vi "Configure Channel Trigger.vi"(6 "Trigger Level (0 V)":dbl, 7 "Units (0: Volt)":i32(ring) items=["Volt", "Ampere"], 8 "error in (no error)":errorcluster, 9 "Vertical Range (8.0 V)":dbl=8.0, 10 "Probe Attenuation Factor (1.0 X)":dbl=1.0, 11 "VISA resource name":refnum<visa-resource-name>) -> (0 "error out":errorcluster, 3 "VISA resource name out":refnum<visa-resource-name>)   [LabVIEW 2023, in "Keysight-DSQx3014T.lvlib"]
doc: "Configures the channel setting for External Trigger."
uses:
  Keysight-DSQx3014T.lvlib
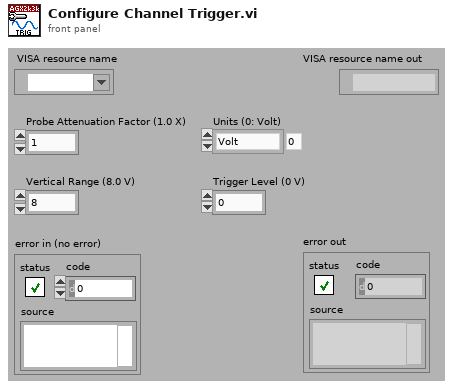
[diagram p1: front panel]
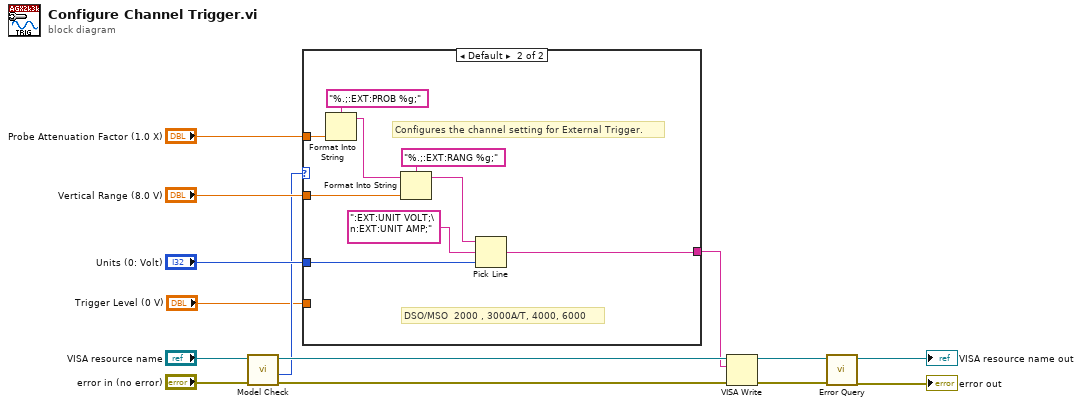
[diagram p0: block diagram]
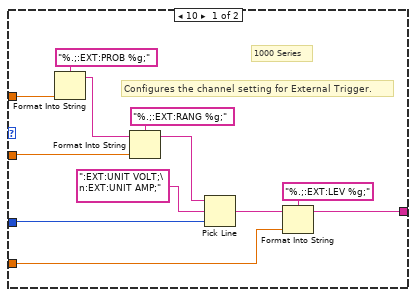
[diagram p2: hidden frame]
diagram:
  n1 = call "Model Check.vi"("error in (no error)"="error in (no error)", "VISA resource name"="VISA resource name") -> ("error out"=w4:errorcluster, "Model"=w2:i32, "VISA resource name out"=w5:refnum<visa-resource-name>)  [unwired: 6 in, 1 out]
  n2 = case shown="Default" w2 {
    tunnel: "Probe Attenuation Factor (1.0 X)" -> [w21 w34]
    tunnel: "Vertical Range (8.0 V)" -> [w20 w31]
    tunnel: "Units (0: Volt)" -> [w19 w29]
    tunnel: [w16 w27] -> w3
    tunnel: "Trigger Level (0 V)" -> [w18 _]
    frame 10 {
      # "1000 Series"
      # "Configures the channel setting for External Trigger."
      n3 = Format Into String(format string="%.;:EXT:PROB %g;", w21) -> (resulting string=w25:string)  [unwired: 2 in, 1 out]
      n4 = Format Into String(format string="%.;:EXT:RANG %g;", initial string=w25, w20) -> (resulting string=w22:string)  [unwired: 1 in, 1 out]
      n5 = Pick Line(string ("")=w22, multi-line string=":EXT:UNIT VOLT;\n:EXT:UNIT AMP;", line index=w19) -> (output string=w17:string)
      n6 = Format Into String(format string="%.;:EXT:LEV %g;", initial string=w17, w18) -> (resulting string=w16:string)  [unwired: 1 in, 1 out]
    }
    frame Default {
      # "DSO/MSO  2000 , 3000A/T, 4000, 6000"
      # "Configures the channel setting for External Trigger."
      n7 = Format Into String(format string="%.;:EXT:PROB %g;", w34) -> (resulting string=w33:string)  [unwired: 2 in, 1 out]
      n8 = Format Into String(format string="%.;:EXT:RANG %g;", initial string=w33, w31) -> (resulting string=w28:string)  [unwired: 1 in, 1 out]
      n9 = Pick Line(string ("")=w28, multi-line string=":EXT:UNIT VOLT;\n:EXT:UNIT AMP;", line index=w29) -> (output string=w27:string)
    }
  }
  n10 = VISA Write(VISA resource name=w5, write buffer=w3, error in (no error)=w4) -> (VISA resource name out=w11:refnum<visa-resource-name>, error out=w10:errorcluster)  [unwired: 1 out]
  n11 = call "Error Query.vi"("error in (no error)"=w10, "VISA resource name"=w11) -> ("error out"=→"error out":errorcluster, "VISA resource name out"=→"VISA resource name out":refnum<visa-resource-name>)  [unwired: 8 out]
